vi "JAPsubscribeINT(NI).vi"(8 "error in":errorcluster, 11 "JAPCintIN":refnum<class "JSubscribe.lvclass">) -> (0 "error out":errorcluster, 2 "JAPCint":string, 3 "JAPCintOUT":refnum<class "JSubscribe.lvclass">)   [LabVIEW 2014]
uses:
  <userlib>/_RADE/RIO/JAPC/classes/JSubscribe/JSubscribe.lvclass
  <userlib>/_RADE/RIO/JAPC/classes/JSubscribe/JAPCSubscribe.vi
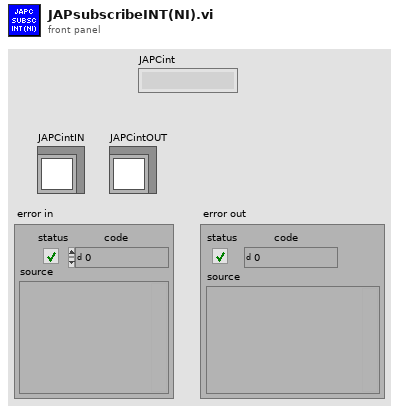
[diagram p1: front panel]
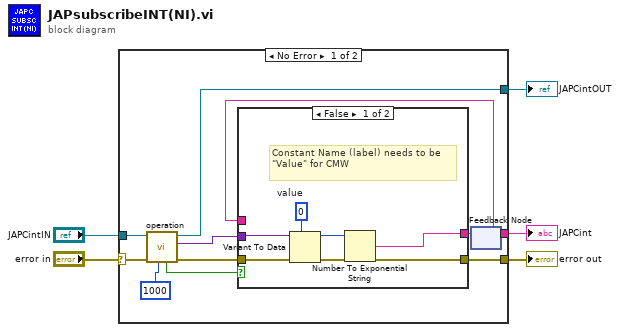
[diagram p0: block diagram]
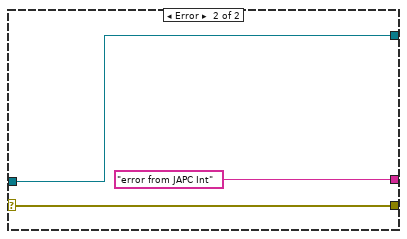
[diagram p3: hidden frame]
diagram:
  n1 = case shown="No Error" "error in" {
    selector: "error in" -> [w10 w26]
    tunnel: [w14 w26] -> w3
    tunnel: "JAPCintIN" -> [w11 w25]
    tunnel: [w8 w25] -> w2
    tunnel: [w6 "error from JAPC Int"] -> w1
    frame No Error {
      n2 = call-poly <userlib>:"operation.vi"("Timeout (10000 ms)"=1000, "error in (no error)"=w10, "Object in"=w11) -> ("error out"=w15:errorcluster, "Data"=w9:variant, "Object out"=w8:refnum<class "JSubscribe.lvclass">, "Timeout?"=w12:bool)  [unwired: 3 in, 2 out]
      n3 = feedback #1() -> (w6:string)  [unwired: 1 in]
      n4 = case shown="False" w12 {
        tunnel: w15 -> [w21 w23]
        tunnel: [w19 w23] -> w14
        tunnel: w9 -> [w20 _]
        tunnel: [w17 w22] -> w7
        tunnel: w6 -> [_ w22]
        frame False {
          w16 = i16 0  # value
          # "Constant Name (label) needs to be \"Value\" for CMW"
          n5 = Variant To Data(error in=w21, type=w16, Variant=w20) -> (data=w18:i16, error out=w19:errorcluster)
          n6 = Number To Exponential String(number=w18) -> (E-format string=w17:string)  [unwired: 3 in]
        }
        frame True {
          # "Subscription Timed Out"
        }
      }
      n7 = feedback-in #1(w7) -> ()
    }
    frame Error {
    }
  }
  "error out" <- w3
  "JAPCintOUT" <- w2
  "JAPCint" <- w1
